vi "rszvl Configure SAN Frequency Center Span.vi"(8 "error in (no error)":errorcluster, 9 "Span":dbl format="%^.3e", 10 "Center Frequency":dbl format="%#.9p", 11 "VISA resource name":refnum<visa-resource-name>) -> (0 "error out":errorcluster, 3 "VISA resource name out":refnum<visa-resource-name>)   [LabVIEW 2014]
doc: "This VI configures the frequency range of the spectrum analyzer using the center frequency and the frequency span. If span corresponds to zero hertz, then the spectrum analyzer is in time-domain. \nNotes:\n\n(1) In auto-coupled mode, RBW, VBW and Sweep time may be affected by this function.\n\nAttribute(s):\nRSZVL_ATTR_FREQUENCY_CENTER\nRSZVL_ATTR_FREQUENCY_SPAN\n\nRemote-control command(s):\n[SENSe<1|2>:]FREQuency:CENTer\n[SENSe<1|2>:]FREQuency:SPAN"
uses:
  Instance           1 49Saved   rszvl Configure SAN Frequency Center Span .vi
  Instance           2 49Saved   rszvl Configure SAN Frequency Center Span .vi
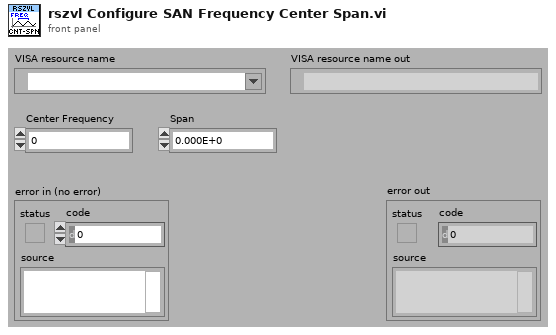
[diagram p1: front panel]
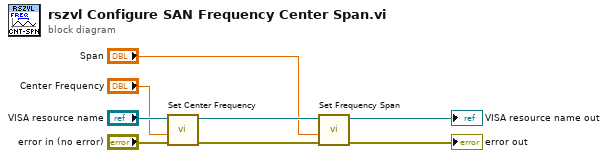
[diagram p0: block diagram]
diagram:
  n1 = call "Set Center Frequency"("error in (no error)"="error in (no error)", "Center Frequency (0.0)"="Center Frequency", "instrument handle"="VISA resource name") -> ("error out"=w6:errorcluster, "instrument handle out"=w5:refnum<visa-resource-name>)  [unwired: 7 in]
  n2 = call "Set Frequency Span"("error in (no error)"=w6, "Frequency Span (0.0)"="Span", "instrument handle"=w5) -> ("error out"=→"error out":errorcluster, "instrument handle out"=→"VISA resource name out":refnum<visa-resource-name>)  [unwired: 7 in]
